vi "DualDigitalOscilloscope.vi"() -> ()   [LabVIEW 2014]
doc: "This digital oscilloscope requires a DAQ device, and can take 2 inputs and display them simultaneously.\n\nSignal input to the ai0 and ai1 portsx will produce a representation of the signals on the front panel. Triggering can be achieved by connecting the function generator's syn/ttl/trig out to the PFI 0 port on the DAQ device\n\nBryan Ghahremani -SID: 1135515\nKenneth Heide -SID: 1269429"
panel:
  out "error out":errorcluster
  in  "Digitizing Parameters":T1={"Number of Samples"=100.0, "Sampling Frequency"=1000.0}
  out "Waveform Graph":dynamicdata(graph)=[{"t0"=timestamp(3496781833.865775 s since 1904-01-01), "dt"=0.001, "Y"=[-2.975625316319028, -2.061001361215725, 0.05032238107267916, 2.0968668469562903, 2.8888497834649045, 2.007115151589184, -0.09137467119722548, -2.1740964557883835, -2.9743102564490957, -1.9469199853989227, 0.19859463779915942, 2.195823798210658, 2.8740556129335393, 1.8923775793383881, -0.24260592755516872, -2.275356027128453, -2.954255593466982, -1.8334961536378251, 0.34752435140335025, 2.2855754090274685, 2.857288884828739, 1.782242601551391, -0.38824826186679445, -2.36773895504637, -2.9269681013260658, -1.7121819859420258, 0.4905362593470927, 2.368423013164574, 2.833289447713146, 1.663231009974999, -0.5352057069525044, -2.4561767103740677, -2.8963929597066675, -1.5875801920741623, 0.6319042833665458, 2.445352899333376, 2.8040298556027934, 1.5455344004228388, -0.6762454525436077, -2.534751523256123, -2.8589137541441767, -1.4613345982648107, 0.7739297614059722, 2.517680114277312, 2.7704963845789323, 1.417974877334712, -0.821559178172693, -2.6070798060159692, -2.8132154250603603, -1.3295000337849292, 0.9116812534121612, 2.5808020244912497, 2.7277576379065507, 1.2877851887891523, -0.9622702506717009, -2.6731615575663574, -2.766859566716238, -1.1976654989952884, 1.0477888615760749, 2.636033678278701, 2.6840326019904066, 1.1562803809504083, -1.0970636059808594, -2.7313529523185993, -2.7135996452986406, -1.0628721173245417, 1.1792937274471962, 2.6879777184456755, 2.6334035999029783, 1.0234604538304422, -1.2364596980418618, -2.7846128740833462, -2.647517892543073, -0.9224897796738273, 1.3121135703780098, 2.7353191092107543, 2.5719255071626472, 0.883736445787423, -1.3679654773077585, -2.8326125574761996, -2.5860388507449272, -0.7863814167145122, 1.4377005814080912, 2.770167625027963, 2.510447394034769, 0.7466424646138489, -1.498156227269697, -2.8723931175082194, -2.508121565335255, -0.6397526466942066, 1.564602570417144, 2.8066599314950347, 2.433846294402653, 0.5996855305697296, -1.6273607096327762, -2.906255908594163, -2.4282316941748685, -0.5016717885249034, 1.6839429767069432, 2.8339469665815793], "attributes"=variant("NI_ChannelName"=variant(string "Voltage"), "NI_UnitDescription"=variant(string "Volts"))}, {"t0"=timestamp(3496781833.865787 s since 1904-01-01), "dt"=0.001, "Y"=[4.934705838327849, 4.934705838327849, 4.937993386804473, 4.937664631960521, 0.0010078684448147255, 0.0010078684448147255, 0.0013366318863368375, 0.0010078684448147255, 4.937993386804473, 4.931418289768797, 4.9320757994872, 4.927801986258674, 0.0013366318863368375, 0.0016653953275384172, 0.0013366318863368375, 0.0013366318863368375, 4.934048328622632, 4.935034593179221, 4.934705838327849, 4.937664631960521, 0.0006791050029721152, 0.0006791050029721152, 0.0010078684448147255, 0.0010078684448147255, 4.938322141647601, 4.937993386804473, 4.9320757994872, 4.932404554345166, 0.0010078684448147255, 0.0013366318863368375, 0.0013366318863368375, 0.0010078684448147255, 4.921884398481721, 4.934377083475653, 4.934377083475653, 4.937007122270143, 0.0013366318863368375, 0.0010078684448147255, 0.0013366318863368375, 0.0010078684448147255, 4.938322141647601, 4.937993386804473, 4.937993386804473, 4.9320757994872, 0.0016653953275384172, 0.0016653953275384172, 0.0013366318863368375, 0.0010078684448147255, 4.921884398481721, 4.9215556435974035, 4.935363348029769, 4.934705838327849, 0.0010078684448147255, 0.0006791050029721152, 0.0010078684448147255, 0.0013366318863368375, 4.939965915850867, 4.937664631960521, 4.937993386804473, 4.934705838327849, 0.0010078684448147255, 0.0006791050029721152, 0.0013366318863368375, 0.0010078684448147255, 4.921884398481721, 4.922213153365216, 4.923528172890963, 4.934377083475653, 0.0010078684448147255, 0.0013366318863368375, 0.0010078684448147255, 0.0016653953275384172, 4.9389796513313815, 4.939308406172035, 4.938322141647601, 4.938650896489904, 0.0016653953275384172, 0.0010078684448147255, 0.0016653953275384172, 0.0016653953275384172, 4.924514437526631, 4.921226888712264, 4.922213153365216, 4.931089534908359, 0.0013366318863368375, 0.0010078684448147255, 0.0010078684448147255, 0.0006791050029721152, 4.937993386804473, 4.939308406172035, 4.937664631960521, 4.938322141647601, 0.0013366318863368375, 0.0013366318863368375, 0.0013366318863368375, 0.0013366318863368375, 4.925171947279627, 4.924185682648899, 4.9215556435974035, 4.921884398481721], "attributes"=variant("NI_ChannelName"=variant(string "Voltage_0"), "NI_UnitDescription"=variant(string "Volts"))}]
  in  "stop":bool
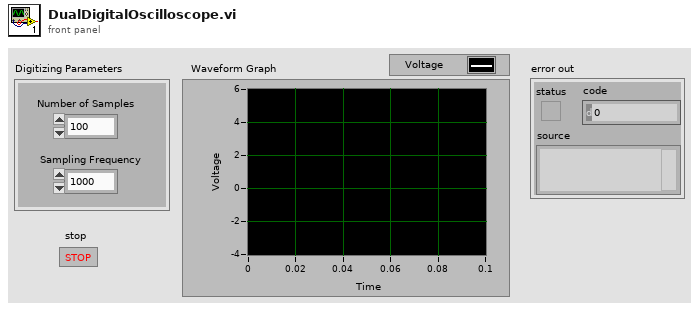
[diagram p1: front panel]
types:
  T1 = cluster{"Number of Samples":dbl, "Sampling Frequency":dbl}
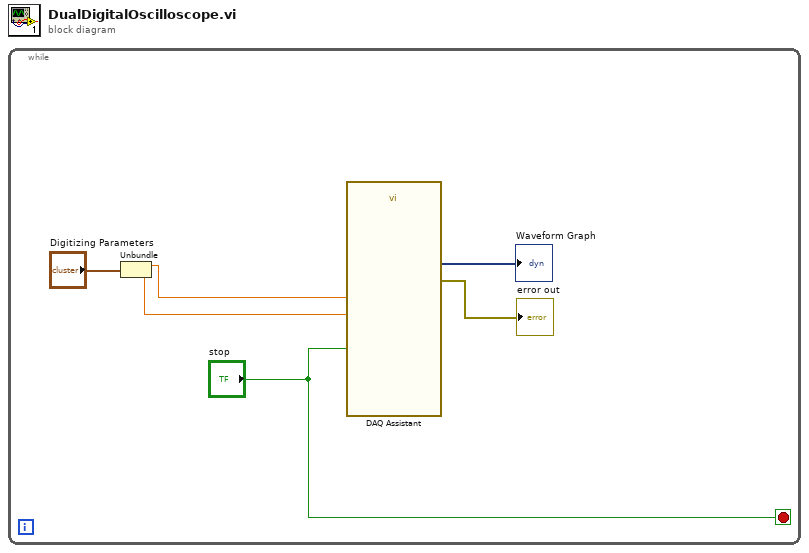
[diagram p0: block diagram]
diagram:
  n1 = while {
    stop <- "stop" stop-if-true
    n2 = Unbundle("Digitizing Parameters") -> ("Number of Samples"=w5:dbl, "Sampling Frequency"=w4:dbl)
    n3 = call "DAQ Assistant"("rate"=w4, "number of samples"=w5, "stop (T)"="stop") -> ("data"=→"Waveform Graph":dynamicdata, "error out"=→"error out":errorcluster)  [unwired: 14 in, 1 out]
  }
